vi "FGV_Channel_Cluster.vi"(8 "error in":errorcluster={"status"=FALSE, "code"=0, "source"="\n"}, 10 "Action":T2, 11 "Channel_Cluster_Array IN":T1 {"Filter" items=["447/60", "475/35", "525/50", "600/37", "647/57", "647LP"]; "Exposure time (s)" min=0.0 max=5.0 step=0.01; "Power (%)" max=100 step=1}) -> (0 "error out":errorcluster, 3 "Channel_Cluster_Array OUT":T1=[{"Laser"=enum."488 nm", "Power (%)"=90, "Exposure time (s)"=0.05, "Channel ON-OFF"=TRUE, "Polar ON-OFF"=TRUE, "Filter"=2}, {"Laser"=enum."561 nm", "Power (%)"=50, "Exposure time (s)"=0.07, "Channel ON-OFF"=TRUE, "Polar ON-OFF"=TRUE, "Filter"=3}, {"Laser"=enum."561 nm", "Power (%)"=30, "Exposure time (s)"=0.09, "Channel ON-OFF"=FALSE, "Polar ON-OFF"=FALSE, "Filter"=3}] {"Filter" items=["447/60", "475/35", "525/50", "600/37", "647/57", "647LP"]; "Exposure time (s)" min=0.0 max=5.0 step=0.01; "Power (%)" max=100 step=1})   [LabVIEW 2026]
doc: "Functional Global Variable:\n- Write the value into the memory \nor\n- Read the value from the memory"
uses:
  TypeDef_FGV.ctl
  TypeDef_Array_ChannelCluster.ctl
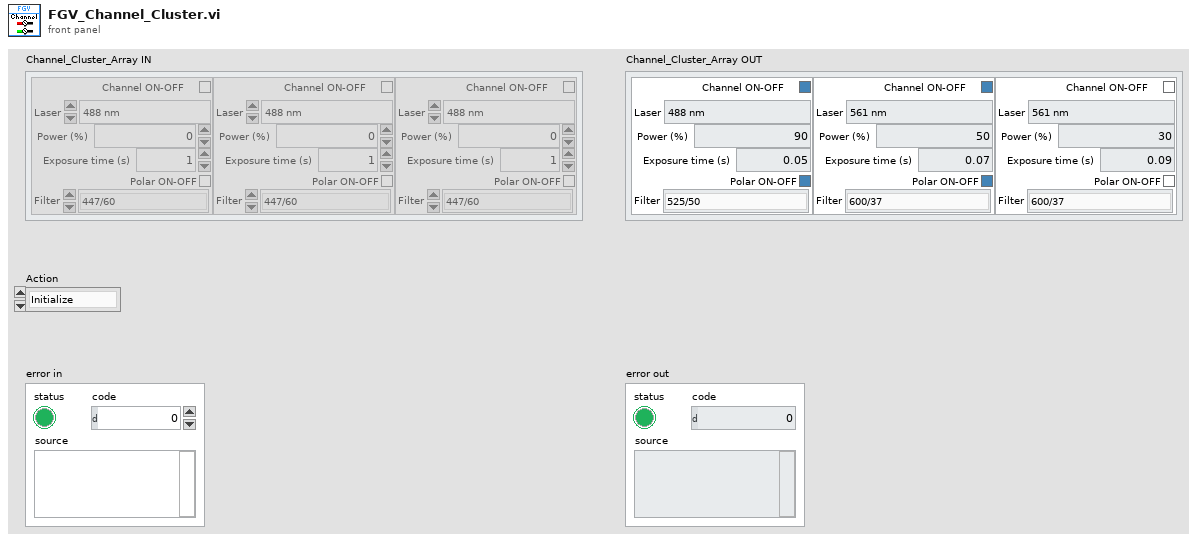
[diagram p1: front panel]
types:
  T1 = typedef "TypeDef_Array_ChannelCluster.ctl" = cluster{"Laser":enum16{"405 nm", "455 nm", "488 nm", "561 nm", "640 nm"}, "Power (%)":u8, "Exposure time (s)":dbl, "Channel ON-OFF":bool, "Polar ON-OFF":bool, "Filter":u16}[]
  T2 = typedef "TypeDef_FGV.ctl" = enum16{"Initialize", "Write", "Read", "Read_File", "Write_to_File"}
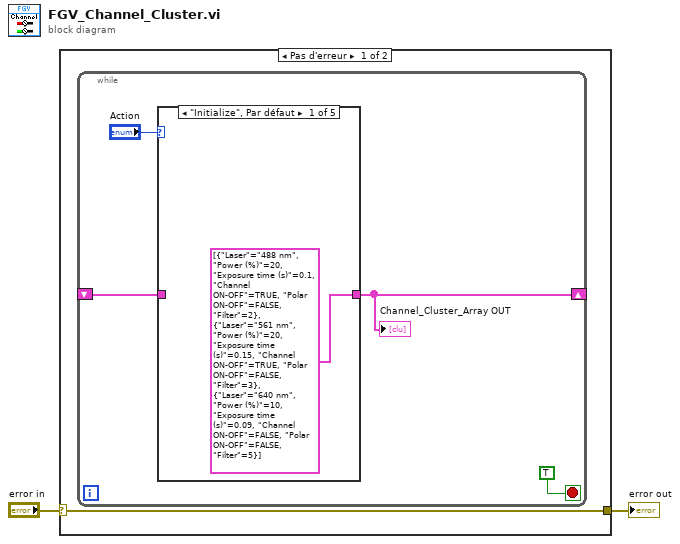
[diagram p0: block diagram]
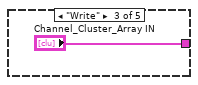
[diagram p3: hidden frame]
diagram:
  n1 = case shown="Pas d'erreur" "error in" {
    selector: "error in" -> [w3 w13]
    tunnel: [w3 w13] -> w1
    frame No Error {
      n2 = while {
        shift-right: [w4] -> _
        shift-left: _ -> [w5]
        stop <- TRUE stop-if-true
        n3 = case shown="\"Initialize\", Par défaut" "Action" {
          tunnel: w5 -> [_ w9 _ w11 w12]
          tunnel: [T1 [{"Laser"=enum."488 nm", "Power (%)"=20, "Exposure time (s)"=0.1, "Channel ON-OFF"=TRUE, "Polar ON-OFF"=FALSE, "Filter"=2}, {"Laser"=enum."561 nm", "Power (%)"=20, "Exposure time (s)"=0.15, "Channel ON-OFF"=TRUE, "Polar ON-OFF"=FALSE, "Filter"=3}, {"Laser"=enum."640 nm", "Power (%)"=10, "Exposure time (s)"=0.09, "Channel ON-OFF"=FALSE, "Polar ON-OFF"=FALSE, "Filter"=5}] ("Channel_Cluster_Array OUT") w9 "Channel_Cluster_Array IN" w11 w12] -> w4
          frame "Initialize", Default {
          }
          frame "Read" {
          }
          frame "Write" {
          }
          frame "Read_File" {
            # "A FAIRE"
          }
          frame "Write_to_File" {
            # "A Faire"
          }
        }
        "Channel_Cluster_Array OUT" <- w4
      }
    }
    frame Error {
    }
  }
  "error out" <- w1
